vi "RemoveAllButNFrames.vi"(10 "Laser to delete (BGR)":dbl, 11 "Array":dbl[][](array[numeric])) -> (3 "Array 2":dbl[][](array[numeric]))   [LabVIEW 2015]
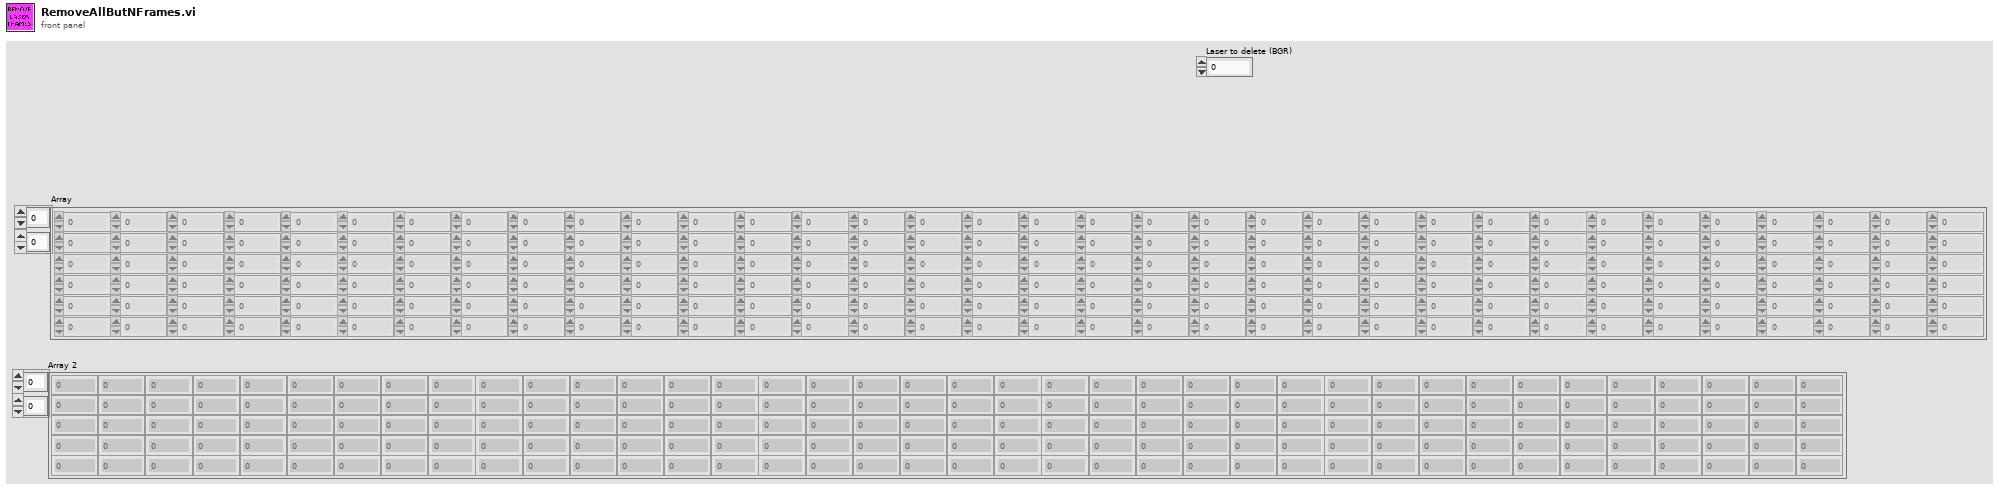
[diagram p1: front panel]
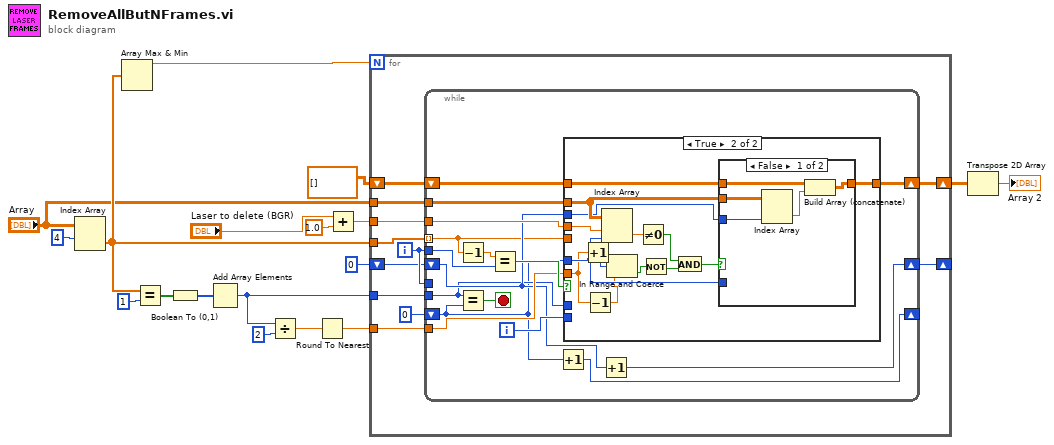
[diagram p0: block diagram]
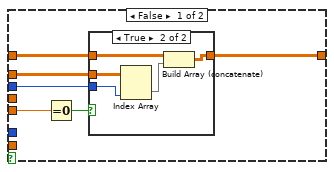
[diagram p2: hidden frame]
diagram:
  n1 = Index Array(array="Array", index (row)=4) -> (element=w13:dbl[])  [unwired: 1 in]
  n2 = Array Max & Min(array=w13) -> (max value=w14:dbl)  [unwired: 3 out]
  n3 = Equal?(x=w13, y=1 ("index (row)")) -> (x = y?=w16:bool[])
  n4 = Boolean To (0,1)(Boolean=w16) -> (0, 1=w15:i16[])
  n5 = Add Array Elements(numeric array=w15) -> (sum=w9:i16)
  n6 = Divide(x=w9, y=i16 2) -> (x/y=w7:dbl)
  n7 = Round To Nearest(number=w7) -> (nearest integer value=w6:dbl)
  n8 = Add(x="Laser to delete (BGR)", y=1.0) -> (x+y=w10:dbl)
  n9 = for {
    N: w14 -> [_]
    tunnel: w9 -> [w29]
    tunnel: w13 -> [w28]
    tunnel: w10 -> [w26]
    tunnel: w6 -> [w25]
    tunnel: "Array" -> [w24]
    shift-right: [w23] -> w2
    shift-left: dbl[][] [] ("Array") -> [w22]
    shift-right: [w19] -> _
    shift-left: 0 ("index (row)") -> [w20]
    i -> [w21]
    n10 = while {
      tunnel: w29 -> [w33]
      tunnel: w28 -> [w34] mode=indexing
      tunnel: w21 -> [w45]
      shift-right: [w30] -> _
      shift-left: 0 ("index (row)") -> [w32]
      tunnel: w26 -> [w43]
      tunnel: w25 -> [w42]
      tunnel: w24 -> [w41]
      tunnel: w21 -> [_]
      shift-right: [w39] -> w23
      shift-left: w22 -> [w38]
      shift-right: [w37] -> w19
      shift-left: w20 -> [w36]
      i -> [w40]
      stop <- w31 stop-if-true
      n11 = Decrement(x=w34) -> (x-1=w35:dbl)
      n12 = Equal?(x=w33, y=w32) -> (x = y?=w31:bool)
      n13 = Equal?(x=w35, y=w45) -> (x = y?=w44:bool)
      n14 = Increment(x=w32) -> (x+1=w30:i32)
      n15 = case shown="True" w44 {
        tunnel: w32 -> [_ w62]
        tunnel: w41 -> [w46 w67]
        tunnel: w43 -> [_ w71]
        tunnel: w33 -> [_ _]
        tunnel: w42 -> [_ w60]
        tunnel: [w48 w66] -> w39
        tunnel: w40 -> [_ _]
        tunnel: w38 -> [w49 w65]
        tunnel: w36 -> [w47 w64]
        tunnel: w34 -> [w51 _]
        frame False {
          n16 = Equal To 0?(x=w51) -> (x = 0?=w50:bool)
          n17 = case shown="True" w50 {
            tunnel: w49 -> [w52 w57]
            tunnel: [w52 w56] -> w48
            tunnel: w47 -> [_ w55]
            tunnel: w46 -> [_ w54]
            frame False {
            }
            frame True {
              n18 = Index Array(array=w54, index (col)=w55) -> (element=w53:dbl[])  [unwired: 1 in]
              n19 = Build Array (concatenate)(w57, w53) -> (w56:dbl[][])
            }
          }
        }
        frame True {
          n20 = Increment(x=w60) -> (x+1=w58:dbl)
          n21 = Decrement(x=w60) -> (x-1=w61:dbl)
          n22 = Index Array(array=w67, index (row)=w71, index (col)=w62) -> (element=w70:dbl)
          n23 = In Range and Coerce(upper limit=w58, x=w62, lower limit=w61) -> (In Range?=w68:bool)  [unwired: 1 out]
          n24 = Not Equal To 0?(x=w70) -> (x != 0?=w69:bool)
          n25 = Not(x=w68) -> (.not. x?=w59:bool)
          n26 = And(x=w69, y=w59) -> (x .and. y?=w63:bool)
          n27 = case shown="False" w63 {
            tunnel: w67 -> [w75 _]
            tunnel: w62 -> [_ _]
            tunnel: [w76 w77] -> w66
            tunnel: w64 -> [w74 _]
            tunnel: w65 -> [w72 w77]
            frame False {
              n28 = Index Array(array=w75, index (col)=w74) -> (element=w73:dbl[])  [unwired: 1 in]
              n29 = Build Array (concatenate)(w72, w73) -> (w76:dbl[][])
            }
            frame True {
            }
          }
        }
      }
      n30 = Increment(x=w36) -> (x+1=w37:i32)
    }
  }
  n31 = Transpose 2D Array(2D array=w2) -> (transposed array=→"Array 2":dbl[][])
